vi "UI.vi"(8 "error in":errorcluster) -> (0 "error out":errorcluster)   [LabVIEW 2020, in "AR Example.lvlib" / "UI.lvclass"]
uses:
  UI.lvclass
  UI.lvclass/UI.ctl
  5c043f1d-1f0f-4328-be52-318364ab5adb.vi
  g_ar_toolkit.image/DrawImageToPictureARGB.vi
  g_ar_toolkit.image/DrawImageToPictureARGB.vi/8cd07b1b-062e-4fe4-9e87-2eb3dc89fe0e.vi
  g_ar_toolkit.common/Module Path.vi
  <vilib>/Utility/error.llb/Error Cluster From Error Code.vi
  App/App.lvclass
  g_ar_toolkit.image/g_ar_toolkit.image.lvlib
panel:
  out "3D Picture":refnum<vi>(3d-picture)
  out "Tab Control":T1(tab)
  in  "ConfigDirectory":path caption="Camera Configuration Directory"
  in  "Load Config":bool
  out "Summary":string
  in  "FileList":i32(listbox) caption="Choose a Camera Configuration File to Load..."
  in  "New Camera Config":bool
  in  "Camera Format":i32(ring) caption="Format" items=["320 x 180 (FPS 15)", "320 x 180 (FPS 30)", "320 x 240 (FPS 15)", "320 x 240 (FPS 30)", "352 x 288 (FPS 15)", "352 x 288 (FPS 30)", "424 x 240 (FPS 15)", "424 x 240 (FPS 30)", "640 x 360 (FPS 15)", "640 x 360 (FPS 30)", "640 x 480 (FPS 15)", "640 x 480 (FPS 30)", "848 x 480 (FPS 15)", "848 x 480 (FPS 20)", "848 x 480 (FPS 30)", "960 x 540 (FPS 15)", "960 x 540 (FPS 30)", "1280 x 720 (FPS 10)", "1280 x 720 (FPS 15)", "1280 x 720 (FPS 30)"]
  in  "Cancel Camera Setup":bool
  out "Preview":picture
  in  "Start Camera Calibration":bool
  in  "Enumerate":bool
  in  "Camera Source":i32(ring) caption="Source" items=["Integrated Camera"]
  in  "Start/Stop Preview":bool
  # "Choose File to Load"
  # "Tag Setup and Print"
  # "Map Markers? or do it live?"
  # "Show/Print Board"
  # "show help gif"
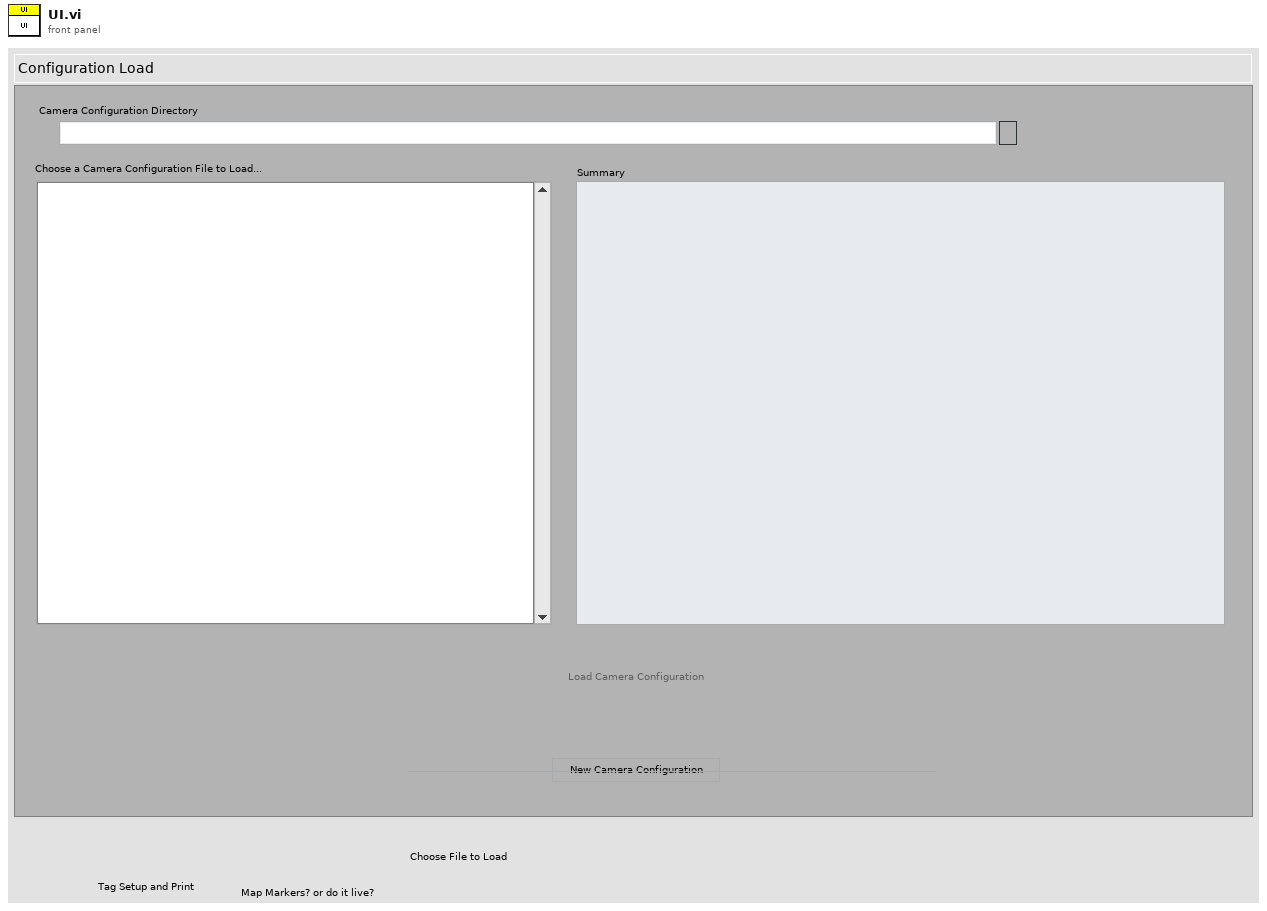
[diagram p1: front panel]
types:
  T1 = enum32{"Configuration Load", "Camera Setup", "Camera Calibration"}
  T2 = enum16{"Reinit Defaults", "Global", "Config", "Setup"}
  T3 = enum16{"Reinit Defaults", "Global", "Config", "Setup"}[]
  T4 = typedef "AR Example.lvlib/UI.lvclass/Event Registration.ctl" = refnum<event-registration>
  T5 = typedef "g_ar_toolkit.image.lvlib/Image Draw Offset.ctl" = cluster{"Top":i16, "Left":i16}
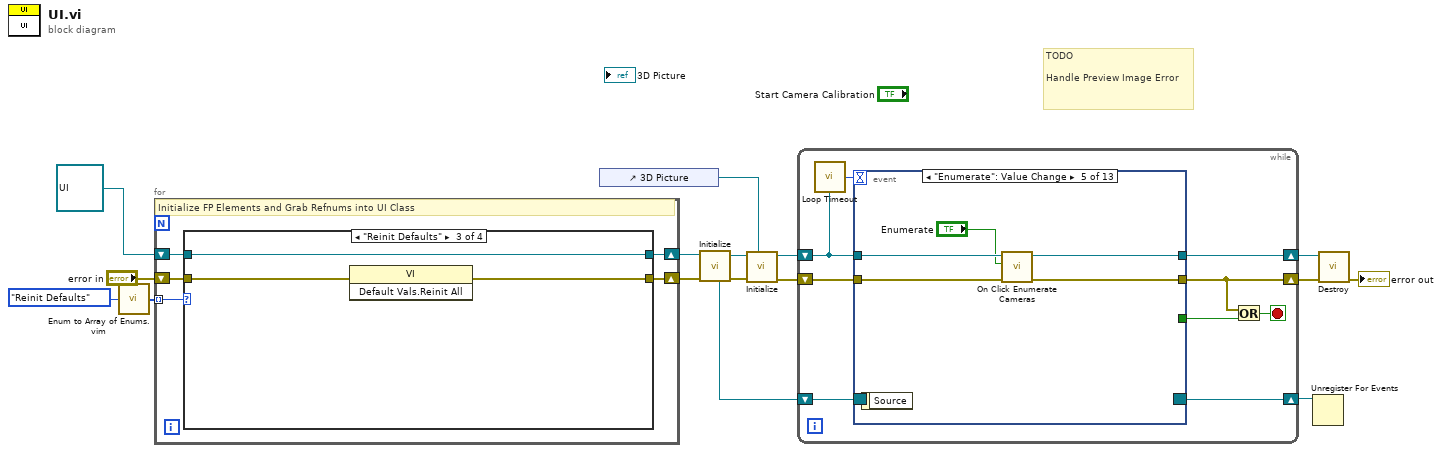
[diagram p0: block diagram]
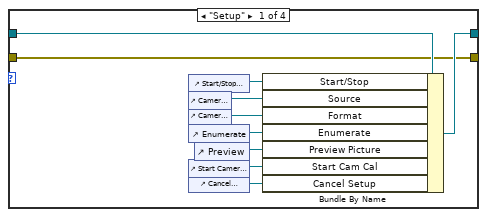
[diagram p2: hidden frame]
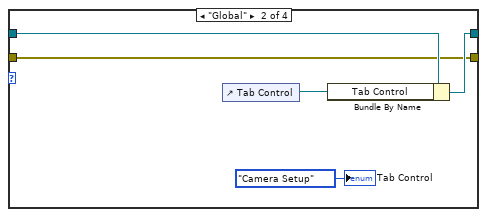
[diagram p3: hidden frame]
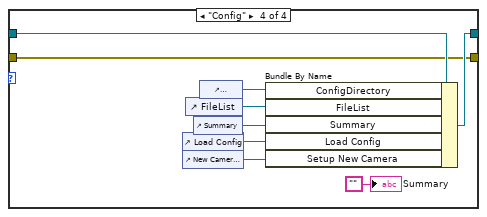
[diagram p4: hidden frame]
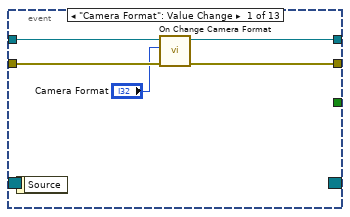
[diagram p5: hidden frame]
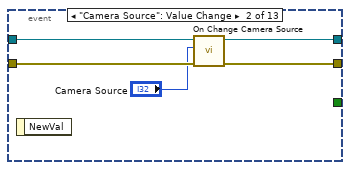
[diagram p6: hidden frame]
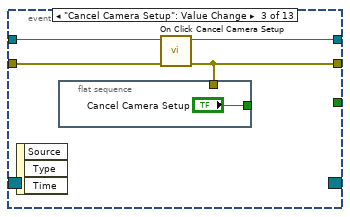
[diagram p7: hidden frame]
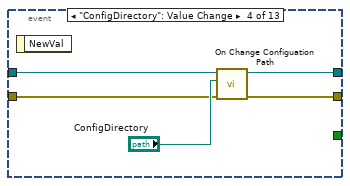
[diagram p8: hidden frame]
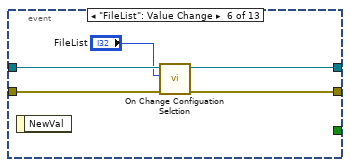
[diagram p9: hidden frame]
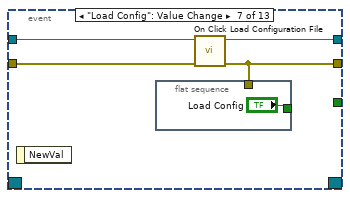
[diagram p10: hidden frame]
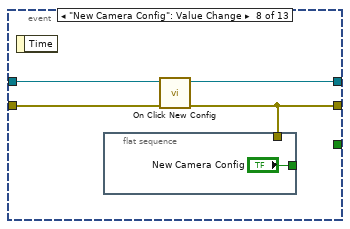
[diagram p11: hidden frame]
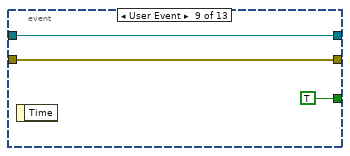
[diagram p12: hidden frame]
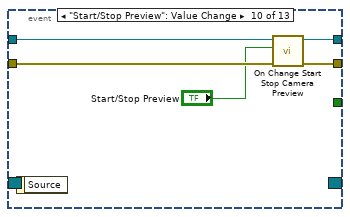
[diagram p13: hidden frame]
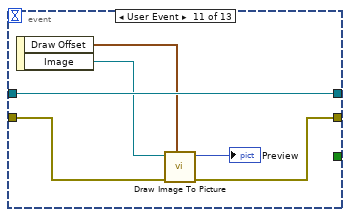
[diagram p14: hidden frame]
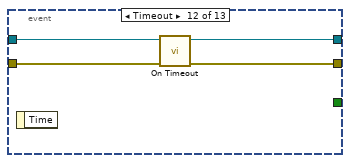
[diagram p15: hidden frame]
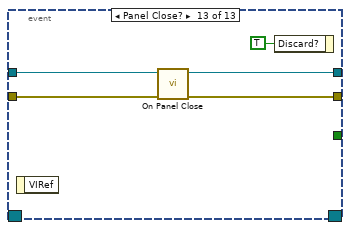
[diagram p16: hidden frame]
diagram:
  # "TODO\n\nHandle Preview Image Error"
  n1 = call "Enum to Array of Enums.vim"("enum"=T2."Reinit Defaults") -> ("array of enums"=w14:T3)
  n2 = for {
    shift-right: [w20] -> w8
    shift-left: refnum<class "UI.lvclass"> refnum ("AR Example.lvlib:UI.lvclass") -> [w21]
    tunnel: w14 -> [w19] mode=indexing
    shift-right: [w18] -> w9
    shift-left: "error in" -> [w17]
    # "Initialize FP Elements and Grab Refnums into UI Class"
    n3 = case shown="\"Reinit Defaults\"" w19 {
      tunnel: w21 -> [w31 w36 w38 w48]
      tunnel: [w30 w35 w38 w47] -> w20
      tunnel: [w25 w33 w37 w41] -> w18
      tunnel: w17 -> [w25 w33 w39 w41]
      frame "Setup" {
        n4 = control-ref of="Start/Stop Preview"() -> (w29:refnum<vi>)
        n5 = control-ref of="Camera Source"() -> (w23:refnum<vi>)
        n6 = control-ref of="Camera Format"() -> (w22:refnum<vi>)
        n7 = control-ref of="Enumerate"() -> (w28:refnum<vi>)
        n8 = control-ref of="Start Camera Calibration"() -> (w26:refnum<vi>)
        n9 = control-ref of="Cancel Camera Setup"() -> (w24:refnum<vi>)
        n10 = control-ref of="Preview"() -> (w27:refnum<vi>)
        n11 = Bundle By Name(cluster=w31, "Start/Stop"=w29, "Source"=w23, "Format"=w22, "Enumerate"=w28, "Preview Picture"=w27, "Start Cam Cal"=w26, "Cancel Setup"=w24) -> (w30:refnum<class "UI.lvclass">)
      }
      frame "Global" {
        n12 = control-ref of="Tab Control"() -> (w34:refnum<vi>)
        n13 = Bundle By Name(cluster=w36, "Tab Control"=w34) -> (w35:refnum<class "UI.lvclass">)
        "Tab Control" <- T1."Camera Setup" ("Tab Control")
      }
      frame "Reinit Defaults" {
        n14 = invoke class="VI" method="Default Vals.Reinit All"(error in=w39) -> (error out=w37:errorcluster)  [unwired: 2 in, 2 out]
      }
      frame "Config" {
        n15 = control-ref of="Load Config"() -> (w43:refnum<vi>)
        n16 = control-ref of="New Camera Config"() -> (w42:refnum<vi>)
        n17 = control-ref of="FileList"() -> (w45:refnum<vi>)
        n18 = control-ref of="Summary"() -> (w44:refnum<vi>)
        n19 = control-ref of="ConfigDirectory"() -> (w46:refnum<vi>)
        n20 = Bundle By Name(cluster=w48, "ConfigDirectory"=w46, "FileList"=w45, "Summary"=w44, "Load Config"=w43, "Setup New Camera"=w42) -> (w47:refnum<class "UI.lvclass">)
        "Summary" <- "" ("Summary")
      }
    }
  }
  n21 = control-ref of="3D Picture"() -> (w11:refnum<vi>)
  n22 = call "Initialize.vi"("error in (no error)"=w9, "UI in"=w8) -> ("error out"=w7:errorcluster, "UI out"=w6:refnum<class "UI.lvclass">, "Event Registration Refnum"=w5:T4)  [unwired: 7 in]
  n23 = call "Initialize.vi"("3D Picture Refnum"=w11, "error in"=w7, "AR Example.lvlib:UI.lvclass"=w6) -> ("error out"=w12:errorcluster, "App out"=w13:refnum<class "App.lvclass">)  [unwired: 7 in]
  n24 = while {
    shift-right: [w56] -> w3
    shift-left: w13 -> [w49]
    shift-right: [w54] -> w2
    shift-left: w12 -> [w57]
    shift-right: [w52] -> w4
    shift-left: w5 -> [w53]
    stop <- w55 stop-if-true
    n25 = call "Loop Timeout.vi"("App in"=w49) -> ("Timeout"=w50:i32)
    n26 = event shown="[4] \"Enumerate\": Value Change" {
      selector: w53 -> [_ _ _ _ _ _ _ _ _ _ _ _ _]
      dyn-events: [_ _ _ _ _ _ _ _ _ _ _ _ _] -> w52
      timeout: w50 -> [_ _ _ _ _ _ _ _ _ _ _ _ _]
      tunnel: w49 -> [w60 w67 w71 w77 w80 w85 w91 w95 w100 w103 w111 w113 w120]
      tunnel: w57 -> [w62 w66 w70 w75 w82 w87 w90 w96 w99 w105 w110 w115 w117]
      tunnel: [w59 w65 w69 w74 w79 w84 w89 w94 w100 w102 w111 w112 w119] -> w56
      tunnel: [w61 w64 w68 w73 w81 w86 w88 w93 w99 w104 w109 w114 w118] -> w54
      tunnel: [_ _ _ _ _ _ _ _ TRUE _ _ _ _] -> w51
      event "Camera Format": Value Change {
        n27 = event-data() -> ()  [unwired: 1 in, 1 out]
        n28 = call "On Change Camera Format.vi"("error in (no error)"=w62, "Selection"="Camera Format", "App in"=w60) -> ("error out"=w61:errorcluster, "App out"=w59:refnum<class "App.lvclass">)  [unwired: 7 in]
      }
      event "Camera Source": Value Change {
        n29 = event-data() -> ()  [unwired: 1 in, 1 out]
        n30 = call "On Change Camera Source.vi"("error in (no error)"=w66, "Selection"="Camera Source", "App in"=w67) -> ("error out"=w64:errorcluster, "App out"=w65:refnum<class "App.lvclass">)  [unwired: 7 in]
      }
      event "Cancel Camera Setup": Value Change {
        n31 = event-data() -> ()  [unwired: 1 in, 3 out]
        n32 = flat-sequence {
          tunnel: ["Cancel Camera Setup"] -> _
          tunnel: w68 -> [_]
          frame #0 {
          }
        }
        n33 = call "On Click Cancel Camera Setup.vi"("error in (no error)"=w70, "App in"=w71) -> ("error out"=w68:errorcluster, "App out"=w69:refnum<class "App.lvclass">)  [unwired: 8 in]
      }
      event "ConfigDirectory": Value Change {
        n34 = event-data() -> ()  [unwired: 1 in, 1 out]
        n35 = call "On Change Configuation Path.vi"("error in (no error)"=w75, "Path"="ConfigDirectory", "App in"=w77) -> ("error out"=w73:errorcluster, "App out"=w74:refnum<class "App.lvclass">)  [unwired: 7 in]
      }
      event "Enumerate": Value Change {
        n36 = event-data() -> ()  [unwired: 1 in, 1 out]
        n37 = call "On Click Enumerate Cameras.vi"("error in (no error)"=w82, "Value"="Enumerate", "App in"=w80) -> ("error out"=w81:errorcluster, "App out"=w79:refnum<class "App.lvclass">)  [unwired: 7 in]
      }
      event "FileList": Value Change {
        n38 = event-data() -> ()  [unwired: 1 in, 1 out]
        n39 = call "On Change Configuation Selction.vi"("error in (no error)"=w87, "Selection"="FileList", "App in"=w85) -> ("error out"=w86:errorcluster, "App out"=w84:refnum<class "App.lvclass">)  [unwired: 7 in]
      }
      event "Load Config": Value Change {
        n40 = event-data() -> ()  [unwired: 1 in, 1 out]
        n41 = flat-sequence {
          tunnel: ["Load Config"] -> _
          tunnel: w88 -> [_]
          frame #0 {
          }
        }
        n42 = call "On Click Load Configuration File.vi"("error in (no error)"=w90, "App in"=w91) -> ("error out"=w88:errorcluster, "App out"=w89:refnum<class "App.lvclass">)  [unwired: 8 in]
      }
      event "New Camera Config": Value Change {
        n43 = event-data() -> ()  [unwired: 1 in, 1 out]
        n44 = flat-sequence {
          tunnel: ["New Camera Config"] -> _
          tunnel: w93 -> [_]
          frame #0 {
          }
        }
        n45 = call "On Click New Config.vi"("error in (no error)"=w96, "App in"=w95) -> ("error out"=w93:errorcluster, "App out"=w94:refnum<class "App.lvclass">)  [unwired: 8 in]
      }
      event User Event {
        n46 = event-data() -> ()  [unwired: 1 in, 1 out]
      }
      event "Start/Stop Preview": Value Change {
        n47 = event-data() -> ()  [unwired: 1 in, 1 out]
        n48 = call "On Change Start Stop Camera Preview.vi"("error in (no error)"=w105, "Value"="Start/Stop Preview", "App in"=w103) -> ("error out"=w104:errorcluster, "App out"=w102:refnum<class "App.lvclass">)  [unwired: 7 in]
      }
      event User Event {
        n49 = event-data() -> ("Draw Offset"=w106:T5, "Image"=w107:refnum<data-value>)  [unwired: 1 in]
        n50 = call-poly "Draw Image To Picture.vi"("Image Draw Offset (Default 0,0)"=w106, "error in (no error)"=w110, "ARGB Image Source"=w107) -> ("error out"=w109:errorcluster, "Picture"=→"Preview":picture)  [unwired: 7 in]
      }
      event Timeout {
        n51 = event-data() -> ()  [unwired: 1 in, 1 out]
        n52 = call "On Timeout.vi"("error in (no error)"=w115, "App in"=w113) -> ("error out"=w114:errorcluster, "App out"=w112:refnum<class "App.lvclass">)  [unwired: 8 in]
      }
      event Panel Close? {
        n53 = event-data() -> ()  [unwired: 1 in, 1 out]
        n54 = call "On Panel Close.vi"("error in (no error)"=w117, "App in"=w120) -> ("error out"=w118:errorcluster, "App out"=w119:refnum<class "App.lvclass">)  [unwired: 8 in]
        n55 = event-data("Discard?"=TRUE) -> ()  [unwired: 1 in, 1 out]
      }
    }
    n56 = Or(x=w54, y=w51) -> (x .or. y?=w55:bool)
  }
  n57 = Unregister For Events(event registration refnum=w4) -> ()  [unwired: 1 in, 1 out]
  n58 = call "Destroy.vi"("error in (no error)"=w2, "App in"=w3) -> ("error out"=→"error out":errorcluster)  [unwired: 9 in]
